vi "SD卡读写实验.vi"() -> ()   [LabVIEW 2011]
panel:
  out "字符串":string
  out "Read Success?":bool
  out "Write Success?":bool
  out "SD Size（MBytes）":u32
  out "SD_Type":u16
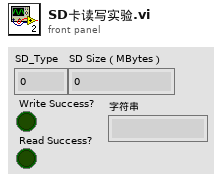
[diagram p1: front panel]
types:
  T1 = enum8{"P0", "P1", "P2", "P3", "P4", "P5", "P6", "P7", "P8", "P9", "P10", "P11", "P12", "P13", "P14", "P15"}
  T2 = enum8{"Port_A", "Port_B", "Port_C", "Port_D", "Port_E", "Port_F", "Port_G"}
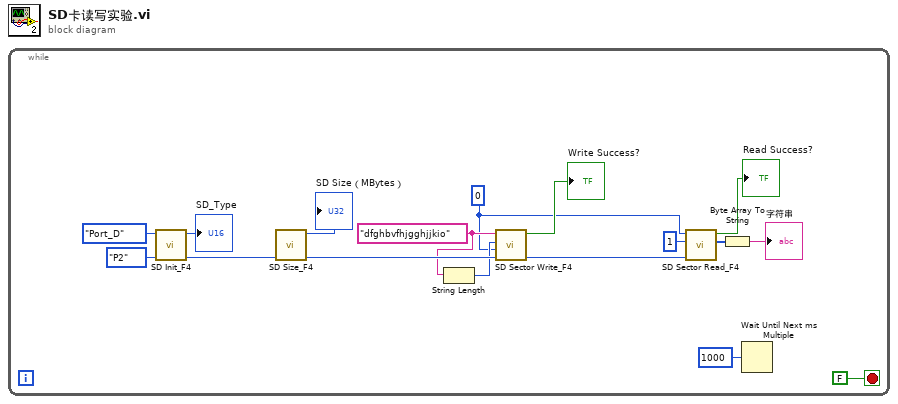
[diagram p0: block diagram]
diagram:
  n1 = while {
    stop <- FALSE stop-if-true
    w7 = u32 0 ("sector_begin")
    w10 = "dfghbvfhjgghjjkio" ("字符串")
    n2 = call <vilib>:"SD Init_F4.vi"("SD_CS_pin"=T1."P2", "SD_CS_PortX"=T2."Port_D") -> ("err_out"=w17:u8, "SD_Type"=→"SD_Type":u16)  [unwired: 8 in]
    n3 = call <vilib>:"SD Size_F4.vi"("err_in"=w17) -> ("err_out"=w16:u8, "SD Size（MBytes）"=→"SD Size（MBytes）":u32)  [unwired: 9 in]
    n4 = String Length(string=w10) -> (length=w11:i32)
    n5 = call <vilib>:"SD Sector Write_F4.vi"("err_in"=w16, "sector_begin"=w7, "String_length"=w11, "字符串"=w10) -> ("err_out"=w8:u8, "Write Success?"=→"Write Success?":bool)  [unwired: 6 in]
    n6 = call <vilib>:"SD Sector Read_F4.vi"("err_in"=w8, "sector_cnt"=u8 1, "sector_begin"=w7) -> ("Sector_Data[cnt*512]"=w4:u8[], "Read Success?"=→"Read Success?":bool)  [unwired: 6 in, 1 out]
    n7 = Byte Array To String(unsigned byte array=w4) -> (string=→"字符串":string)
    n8 = Wait Until Next ms Multiple(millisecond multiple=u32 1000 ("毫秒倍数")) -> ()  [unwired: 1 out]
  }
